vi "DockStaticSubpanels.vi"(8 "ErrorIn":errorcluster, 11 "ReferenceIn":refnum<class "MasterGUI.lvclass">) -> (0 "ErrorOut":errorcluster, 3 "ReferenceIn":refnum<class "MasterGUI.lvclass">)   [LabVIEW 2021, in "MasterGUI.lvclass"]
uses:
  MasterGUI.lvclass
  MasterGUI.lvclass/MasterGUI.ctl
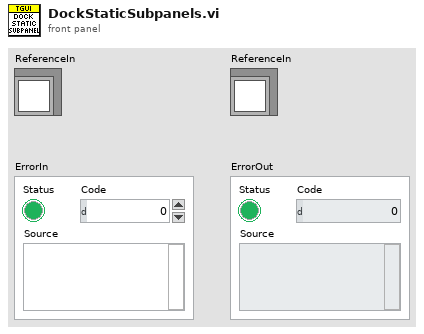
[diagram p1: front panel]
types:
  T1 = typedef "MasterGUI.lvclass/ObjectAttributes.ctl" = cluster{"Interfaces":cluster{"Dummy":refnum<class>}, "Locals":cluster{"MainGUIActive":refnum<queue>, "MainPanel":refnum<vi>, "LayoutPanel":cluster{"PanelVIRef":refnum<vi>, "Labels":string[], "SubPanels":refnum<vi>[]}, "MenuTree":T2[], "Menu":refnum<k9>}, "Persistent":cluster{"StaticDocking":cluster{"ObjectLabel":string, "SubPanelLabel":string}[], "WindowsTitle":string, "AdditionalMenuItems":T2[], "TraceObjectName":string}}
  T2 = typedef "MasterGUI.lvclass/MenuItem.ctl" = cluster{"Parent":string, "Items":string[], "ShortCuts":cluster{"IncludeShiftKey":bool, "IncludeCtrlKey":bool, "ShortcutKey":string}[]}
  T3 = cluster{"ObjectLabel":string, "SubPanelLabel":string}[]
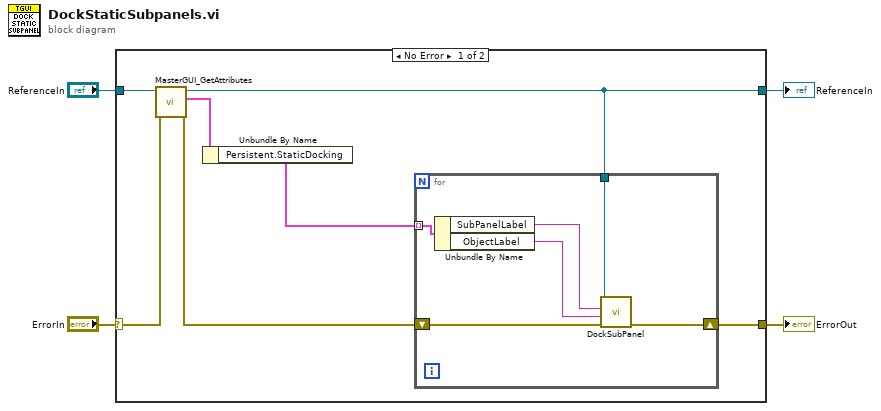
[diagram p0: block diagram]
diagram:
  n1 = case shown="No Error" "ErrorIn" {
    selector: "ErrorIn" -> [w11 w19]
    tunnel: [w9 w19] -> w3
    tunnel: [w5 w18] -> w1
    tunnel: "ReferenceIn" -> [w7 w18]
    frame No Error {
      n2 = call "MasterGUI_GetAttributes.vi"("error in (no error)"=w11, "reference in"=w7) -> ("error out"=w10:errorcluster, "Data"=w8:T1, "reference out"=w5:refnum<class "MasterGUI.lvclass">)  [unwired: 6 in, 1 out]
      n3 = Unbundle By Name(w8) -> ("Persistent.StaticDocking"=w6:T3)
      n4 = for {
        shift-right: [w16] -> w9
        shift-left: w10 -> [w17]
        tunnel: w6 -> [w14] mode=indexing
        tunnel: w5 -> [w15]
        n5 = Unbundle By Name(w14) -> ("SubPanelLabel"=w13:string, "ObjectLabel"=w12:string)
        n6 = call-dynamic "DockSubPanel.vi"("ErrorIn"=w17, "ObjectLabel"=w12, "PanelLabel"=w13, "ReferenceIn"=w15) -> ("ErrorOut"=w16:errorcluster)  [unwired: 6 in, 1 out]
      }
    }
    frame Error {
    }
  }
  "ErrorOut" <- w3
  "ReferenceIn" <- w1
